vi "Visibility.vi"(7 "Visible State":bool, 8 "Error In":errorcluster, 11 "Visible Controls":refnum<vi>[](array[refnum])) -> (0 "Error Out":errorcluster)   [LabVIEW 2018]
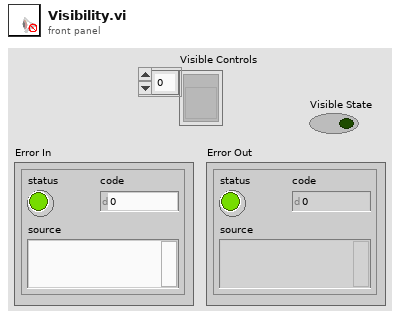
[diagram p1: front panel]
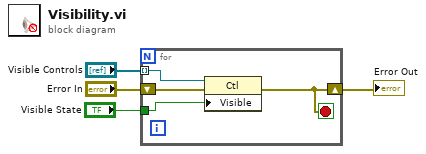
[diagram p0: block diagram]
diagram:
  n1 = for {
    shift-right: [w5] -> w2
    shift-left: "Error In" -> [w7]
    tunnel: "Visible Controls" -> [w8] mode=indexing
    tunnel: "Visible State" -> [w6]
    stop <- w5 stop-if-true
    n2 = property class="Ctl"(reference=w8, error in=w7, "Visible"=w6) -> (error out=w5:errorcluster)  [unwired: 1 out]
  }
  "Error Out" <- w2
